vi "Do Core.vi"(8 "error in (no error)":errorcluster, 9 "Actor in":refnum<class "Actor.lvclass">, 11 "Reply Message":refnum<class "Get Joystick State Msg WFR.lvclass">) -> (0 "error out":errorcluster, 1 "Actor out":refnum<class "Actor.lvclass">, 2 "Reply":variant)   [LabVIEW 2020, in "RPI.SenseHat.Actor.lvlib" / "Get Joystick State Msg WFR.lvclass"]
doc: "(<B>Filename</B>: Actor Framework.lvlib:Reply Msg.lvclass:Do Core.vi)\n\nDefines what an actor does when it receives <B>Reply Message</B>. This method also defines the <B>Reply</B> that is returned to the actor that sent <B>Reply Message</B>.\n\nBy default, this method does nothing, and <B>Reply</B> is the ancestor Message class. A child class must override this method to define behavior and specify a child of the Message class to return in the <B>Reply</B> output."
uses:
  Get Joystick State Msg WFR.lvclass
  <vilib>/ActorFramework/Actor/Actor.lvclass
  RPI.SenseHat.Actor/RPI.SenseHat.Actor.lvclass
  C:/Program Files (x86)/National Instruments/LabVIEW 2020/vi.lib/ActorFramework/Actor/Actor.lvclass
  RPI.SenseHat.Actor/RPI.SenseHat.Actor.lvclass/RPI.SenseHat.Actor.ctl
  03715f3c-f6b0-4b87-b55a-c10d252f7c94.vi
  RPI.SenseHat.Actor/Get Joystick.vi
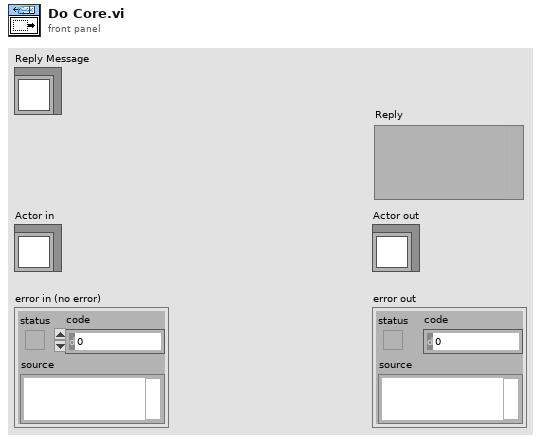
[diagram p1: front panel]
types:
  T1 = typedef "RPI.SenseHat.Joystick.lvlib/Joystick.ctl" = cluster{"Enter":bool, "Down":bool, "Up":bool, "Right":bool, "Left":bool}
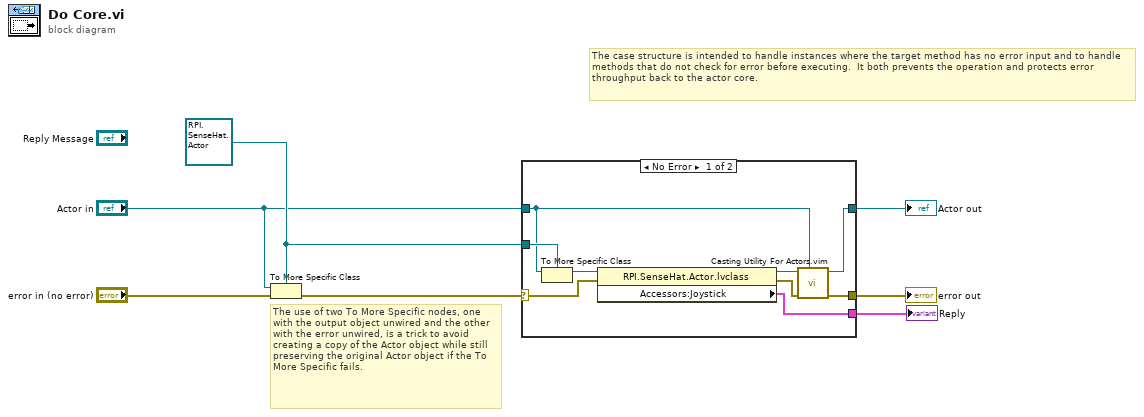
[diagram p0: block diagram]
diagram:
  w6 = refnum<class "RPI.SenseHat.Actor.lvclass"> refnum ("RPI.SenseHat.Actor.lvlib:RPI.SenseHat.Actor.lvclass")
  # "The use of two To More Specific nodes, one with the output object unwired and the other with the error unwired, is a trick to avoid creating a copy of the Actor object while still preserving the original Actor object if the To More Specific fails."
  # "The case structure is intended to handle instances where the target method has no error input and to handle methods that do not check for error before executing.  It both prevents the operation and protects error throughput back to the actor core."
  n1 = To More Specific Class(target class=w6, reference="Actor in", error in="error in (no error)") -> (error out=w7:errorcluster)  [unwired: 1 out]
  n2 = case shown="No Error" w7 {
    selector: w7 -> [w9 w18]
    tunnel: [w13 w18] -> w4
    tunnel: [w14 w17] -> w5
    tunnel: "Actor in" -> [w15 w17]
    tunnel: w6 -> [w16 _]
    tunnel: [w10 _] -> w1
    frame No Error {
      n3 = To More Specific Class(target class=w16, reference=w15) -> (specific class reference=w12:refnum<class "RPI.SenseHat.Actor.lvclass">)  [unwired: 1 in, 1 out]
      n4 = property class="RPI.SenseHat.Actor.lvclass"(reference=w12, error in=w9) -> (reference out=w11:refnum<class "RPI.SenseHat.Actor.lvclass">, error out=w8:errorcluster, "Accessors:Joystick"=w10:T1)
      n5 = call "Casting Utility For Actors.vim"("type"=w15, "error in (no error)"=w8, "Actor in"=w11) -> ("error out"=w13:errorcluster, "Actor out"=w14:refnum<class "Actor.lvclass">)  [unwired: 7 in]
    }
    frame Error {
      # "If type check fails, pass the original object out again."
    }
  }
  "error out" <- w4
  "Actor out" <- w5
  "Reply" <- w1
